vi "plan_to_grbl.vi"(3 "error in (no error)":errorcluster, 5 "Plan GCode":string) -> (0 "error out":errorcluster, 2 "GCode for GRBL":string)   [LabVIEW 2020]
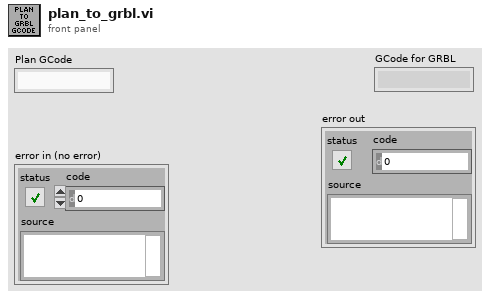
[diagram p1: front panel]
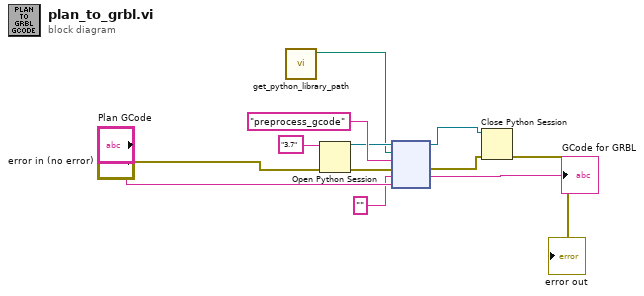
[diagram p0: block diagram]
diagram:
  n1 = call "get_python_library_path.vi"() -> ("Python library path"=w1:path)  [unwired: 11 in]
  n2 = Open Python Session(python version="3.7" ("Python version"), 3:"error in (no error)") -> (session out=w3:refnum<k35>, error out=w5:errorcluster)  [unwired: 1 in]
  n3 = node(w3, w1, "preprocess_gcode" ("function name"), w5, "" ("Python version"), "Plan GCode") -> (w10:refnum<k35>, w11:errorcluster, →"GCode for GRBL":string)  [unwired: 1 in, 2 out]
  n4 = Close Python Session(session in=w10, error in=w11) -> (11:→"error out":errorcluster)
